vi "Rezero ecncoder(SubVI).vi"(7 "Zero":i32, 11 "Encoder":i32) -> (3 "Rezeroed Encoder":i32)   [LabVIEW 2018, in "Elevator.lvlib" / "Elevator Linear.lvclass"]
uses:
  Elevator Linear.lvclass
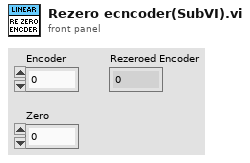
[diagram p1: front panel]
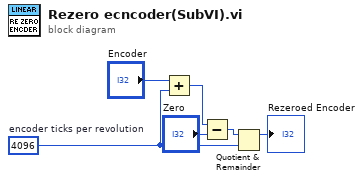
[diagram p0: block diagram]
diagram:
  w5 = 4096  # encoder ticks per revolution
  n1 = Add(x="Encoder", y=w5) -> (x+y=w1:i32)
  n2 = Subtract(x=w1, y="Zero") -> (x-y=w3:i32)
  n3 = Quotient & Remainder(x=w3, y=w5) -> (x-y*floor(x/y)=→"Rezeroed Encoder":i32)  [unwired: 1 out]
